vi "Random2.vi"(1 "Random_num":dbl, 2 "전체횟수":dbl) -> (0 "배열":i32[](array[numeric]))   [LabVIEW 2014]
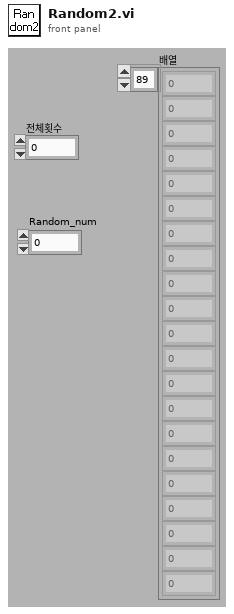
[diagram p1: front panel]
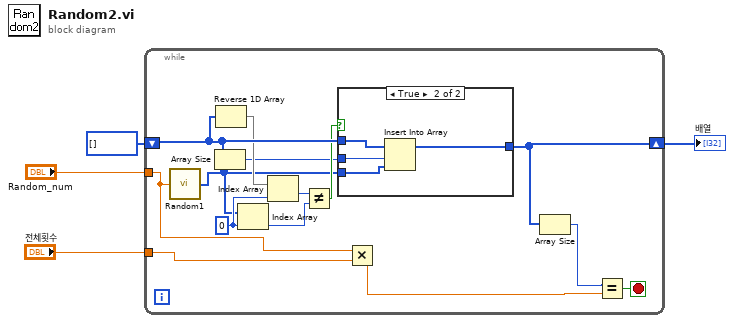
[diagram p0: block diagram]
diagram:
  n1 = while {
    tunnel: "Random_num" -> [w5]
    shift-right: [w17] -> w1
    shift-left: i32[] [] -> [w16]
    tunnel: "전체횟수" -> [w18]
    stop <- w11 stop-if-true
    w7 = 0 ("인덱스")
    n2 = call "Random1.vi"("Random_num"=w5) -> ("배열"=w6:i32[])
    n3 = Array Size(array=w16) -> (size(s)=w8:i32)
    n4 = Reverse 1D Array(array=w16) -> (reversed array=w15:i32[])
    n5 = Index Array(array=w6, index=w7) -> (element=w14:i32)
    n6 = Index Array(array=w15, index=w7) -> (element=w13:i32)
    n7 = Not Equal?(x=w13, y=w14) -> (x != y?=w12:bool)
    n8 = case shown="True" w12 {
      tunnel: w16 -> [w19 w23]
      tunnel: [w19 w22] -> w17
      tunnel: w6 -> [_ w21]
      tunnel: w8 -> [_ w20]
      frame False {
      }
      frame True {
        n9 = Insert Into Array(array=w23, index=w20, new element=w21) -> (w22:i32[])
      }
    }
    n10 = Multiply(x=w5, y=w18) -> (x*y=w9:dbl)
    n11 = Array Size(array=w17) -> (size(s)=w10:i32)
    n12 = Equal?(x=w10, y=w9) -> (x = y?=w11:bool)
  }
  "배열" <- w1
